vi "Send Get SyncData.vi"(7 "Message Priority (Normal)":T1=enum."Normal", 8 "error in (no error)":errorcluster, 11 "Message Enqueuer in":refnum<class "Message Enqueuer.lvclass">) -> (0 "error out":errorcluster, 1 "Theme":refnum<class "Theme.lvclass">, 2 "Data":refnum<class "Data.lvclass">, 3 "Message Enqueuer out":refnum<class "Message Enqueuer.lvclass">)   [LabVIEW 2017, in "Filled Text Fields Actor.lvlib" / "Get SyncData Msg.lvclass"]
uses:
  Get SyncData Msg.lvclass
  <vilib>/ActorFramework/Message Enqueuer/Message Enqueuer.lvclass
  <vilib>/ActorFramework/Message Enqueuer/Message Priority.ctl
  Data/Data.lvclass
  Theme/Theme/Theme.lvclass
  C:/Program Files (x86)/National Instruments/LabVIEW 2017/vi.lib/ActorFramework/Reply Msg/Reply Msg.lvclass
  <vilib>/ActorFramework/Reply Msg/Reply Msg.lvclass/Reply Msg.ctl
  <vilib>/ActorFramework/Message Enqueuer/Message Enqueuer.lvclass/Message Enqueuer.ctl
  <vilib>/ActorFramework/Message Enqueuer/Enqueue.vi
  <vilib>/ActorFramework/Reply Msg/Reply Msg.lvclass
  C:/Program Files (x86)/National Instruments/LabVIEW 2017/vi.lib/ActorFramework/Message/Message.lvclass
  <vilib>/ActorFramework/Message Priority Queue/Priority Enqueue.vi
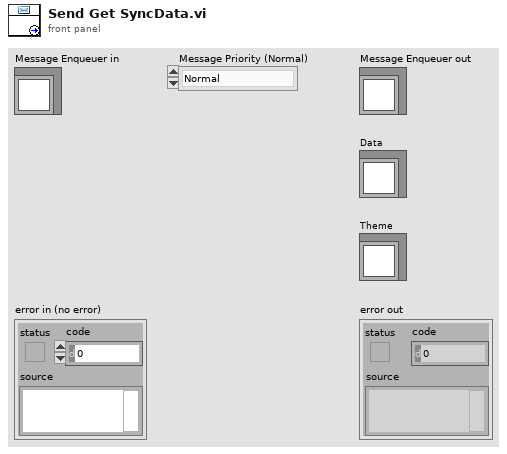
[diagram p1: front panel]
types:
  T1 = typedef "Actor Framework.lvlib/Message Enqueuer.lvclass/Message Priority.ctl" = enum16{"Low", "Normal", "High"}
  T2 = cluster{"Data":refnum<class "Data.lvclass">, "Theme":refnum<class "Theme.lvclass">}
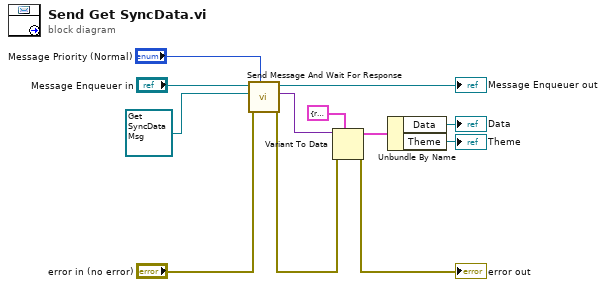
[diagram p0: block diagram]
diagram:
  n1 = call <vilib>:"Send Message And Wait For Response.vi"("Message Priority (Normal)"="Message Priority (Normal)", "error in (no error)"="error in (no error)", "Original Message"=refnum<class "Get SyncData Msg.lvclass"> refnum ("Get SyncData Msg in"), "Message Enqueuer in"="Message Enqueuer in") -> ("error out"=w2:errorcluster, "Reply"=w7:variant, "Message Enqueuer out"=→"Message Enqueuer out":refnum<class "Message Enqueuer.lvclass">)  [unwired: 4 in, 1 out]
  n2 = Variant To Data(error in=w2, type=T2 {"Data"=refnum, "Theme"=refnum} ("cluster"), Variant=w7) -> (data=w5:T2, error out=→"error out":errorcluster)
  n3 = Unbundle By Name(w5) -> ("Data"=→"Data":refnum<class "Data.lvclass">, "Theme"=→"Theme":refnum<class "Theme.lvclass">)
